vi "Set panel size and  place center.vi"(0 "VI引用句柄":refnum<vi>, 1 "Close Reference (false)":bool, 2 "FP.WinOrigin in(H & V)":cluster{"Horizontal":i16, "Vertical":i16}, 5 "Panel Width":i32, 7 "Panel Height":i32, 9 "FP.Origin in(H & V)":cluster{"Horizontal":i16, "Vertical":i16}, 11 "error in (no error)":errorcluster, 12 "Set (false)":bool) -> (4 "Application or VI Refnum":refnum<vi>, 15 "error out":errorcluster)   [LabVIEW 2016]
doc: "This VI is used to set the panel size and plce it in the center of the window current"
uses:
  <vilib>/Utility/miscctls.llb/LVRectTypeDef.ctl
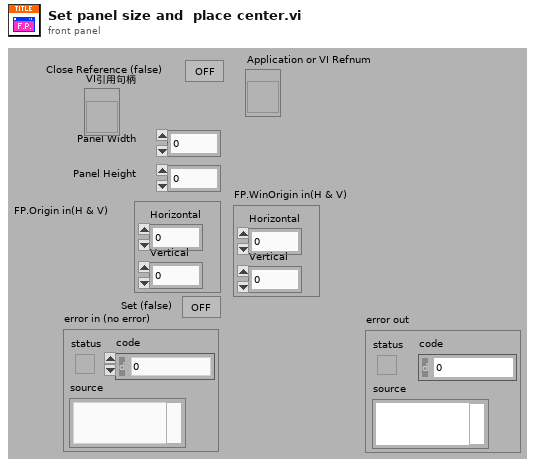
[diagram p1: front panel]
types:
  T1 = typedef "LVRectTypeDef.ctl" = cluster{"Left":i16, "Top":i16, "Right":i16, "Bottom":i16}
  T2 = typedef "LVAllMonitorsDisplayTypeDef.ctl" = cluster{"Bounds":cluster{"Left":i16, "Top":i16, "Right":i16, "Bottom":i16}, "Depth":i16}[]
  T3 = cluster{"Bounds":cluster{"Left":i16, "Top":i16, "Right":i16, "Bottom":i16}, "Depth":i16}
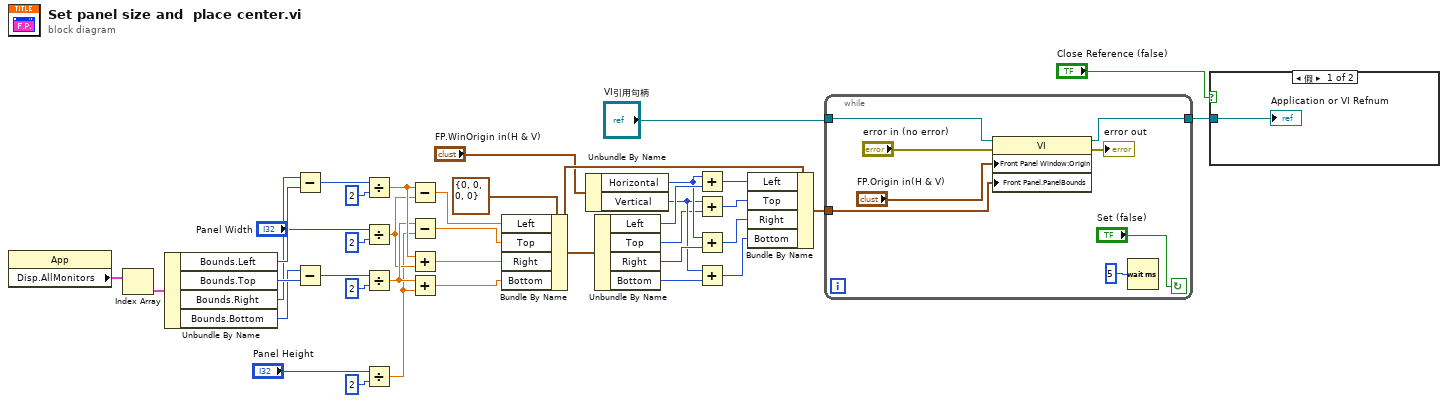
[diagram p0: block diagram]
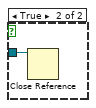
[diagram p2: hidden frame]
diagram:
  n1 = property class="App"() -> ("Disp.AllMonitors"=w16:T2)  [unwired: 2 in, 2 out]
  n2 = Index Array(array=w16) -> (element=w15:T3)  [unwired: 1 in]
  n3 = Unbundle By Name(w15) -> ("Bounds.Left"=w39:i16, "Bounds.Top"=w38:i16, "Bounds.Right"=w37:i16, "Bounds.Bottom"=w36:i16)
  n4 = Subtract(x=w37, y=w39) -> (x-y=w35:i16)
  n5 = Subtract(x=w36, y=w38) -> (x-y=w33:i16)
  n6 = Divide(x=w35, y=i16 2) -> (x/y=w27:dbl)
  n7 = Divide(x="Panel Width", y=2) -> (x/y=w25:dbl)
  n8 = Divide(x=w33, y=i16 2) -> (x/y=w26:dbl)
  n9 = Divide(x="Panel Height", y=2) -> (x/y=w24:dbl)
  n10 = Subtract(x=w27, y=w25) -> (x-y=w23:dbl)
  n11 = Subtract(x=w26, y=w24) -> (x-y=w21:dbl)
  n12 = Add(x=w27, y=w25) -> (x+y=w20:dbl)
  n13 = Add(x=w26, y=w24) -> (x+y=w22:dbl)
  n14 = Bundle By Name(cluster=T1 {"Left"=0, "Top"=0, "Right"=0, "Bottom"=0} ("显示:主工作区"), "Left"=w23, "Top"=w21, "Right"=w20, "Bottom"=w22) -> (w14:T1)
  n15 = Unbundle By Name("FP.WinOrigin in(H & V)") -> ("Horizontal"=w10:i16, "Vertical"=w6:i16)
  n16 = Unbundle By Name(w14) -> ("Left"=w12:i16, "Top"=w3:i16, "Right"=w9:i16, "Bottom"=w5:i16)
  n17 = Add(x=w10, y=w12) -> (x+y=w11:i16)
  n18 = Add(x=w6, y=w3) -> (x+y=w7:i16)
  n19 = Add(x=w10, y=w9) -> (x+y=w8:i16)
  n20 = Add(x=w6, y=w5) -> (x+y=w4:i16)
  n21 = Bundle By Name(cluster=w14, "Left"=w11, "Top"=w7, "Right"=w8, "Bottom"=w4) -> (w2:T1)
  n22 = while {
    tunnel: [w47] -> w18
    tunnel: "VI引用句柄" -> [w46]
    tunnel: w2 -> [w40]
    stop <- "Set (false)" continue-if-true
    n23 = property class="VI"(reference=w46, error in="error in (no error)", "Front Panel Window:Origin"="FP.Origin in(H & V)", "Front Panel.PanelBounds"=w40) -> (reference out=w47:refnum<vi>, error out=→"error out":errorcluster)
    n24 = Wait (ms)(milliseconds to wait=u32 5) -> ()  [unwired: 1 out]
  }
  n25 = case shown="假" "Close Reference (false)" {
    tunnel: w18 -> [w48 w49]
    frame False {
      "Application or VI Refnum" <- w48
    }
    frame True {
      n26 = Close Reference(reference=w49) -> ()  [unwired: 1 in, 1 out]
    }
  }
